vi "Read Event Data.vi"(11 "Event Generated Msg":refnum<class "Abstract Event Message for View.lvclass">) -> (2 "Event Data":refnum<class "Event.lvclass">)   [LabVIEW 2023, in "MVC Actors.lvlib" / "Abstract Event Message for View.lvclass"]
doc: "Reads the <b>Event</b> data from the concrete implementation of the <b>\"Abstract Event Message for View.lvclass\"</b> abstract message sent to <b>View</b>. This method should be called within the concrete <b>\"Do.vi\"</b> method to read the <b>Event</b> data to be used as an argument to the call of the <b>View</b> method designated to handle the corresponding Event."
uses:
  Abstract Event Message for View.lvclass
  Event/Event.lvclass
  Abstract Event Message for View.lvclass/Abstract Event Message for View.ctl
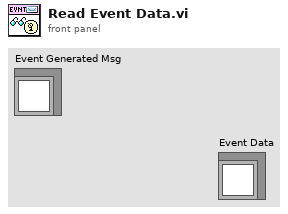
[diagram p1: front panel]
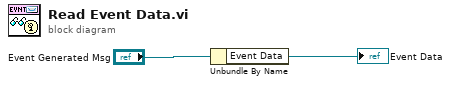
[diagram p0: block diagram]
diagram:
  n1 = Unbundle By Name ("Attribute Unbundler")("Event Generated Msg") -> ("Event Data"=→"Event Data":refnum<class "Event.lvclass">)
